vi "Reserve Coral.vi"(7 "Description":string="Reserve", 8 "Command Info":T1, 10 "Command Name":string) -> (0 "Command Info":T1)   [LabVIEW 2023]
uses:
  <vilib>/Rock Robotics/WPI/Framework/Command Status Info.ctl
  <vilib>/Rock Robotics/WPI/Framework/Completion Status.ctl
  <vilib>/Rock Robotics/WPI/Framework/Completion Notifier.ctl
  Implementation/Coral Setpoints.ctl
  Implementation/Coral Operations.ctl
  Support Code/Teleop Util/Coral States.ctl
  Support Code/Teleop Util/Scoring Levels.ctl
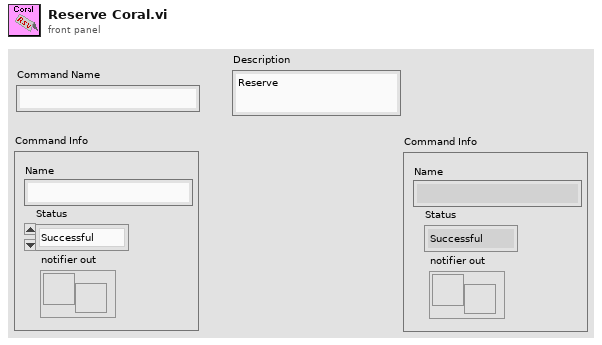
[diagram p1: front panel]
types:
  T1 = typedef "Command Status Info.ctl" = cluster{"Name":string, "Status":T2, "notifier out":T3}
  T2 = typedef "Completion Status.ctl" = enum16{"Successful", "Aborted", "Incomplete"}
  T3 = typedef "Completion Notifier.ctl" = refnum<notifier>
  T4 = typedef "Coral Setpoints.ctl" = cluster{"Operation":T5, "Coral States":T6, "Confirm or Negate":bool, "Positional Array":dbl[], "Setpoint State":T7}
  T5 = typedef "Coral Operations.ctl" = enum16{"Reserve", "Read Current", "Immediate", "Calibrate"}
  T6 = typedef "Coral States.ctl" = enum16{"Grounded", "Coral Intake", "Scoring Sequence", "Hold Position", "Score", "Manual Override", "Climb Safety Mode"}
  T7 = typedef "Scoring Levels.ctl" = enum16{"Trough", "L2", "L3", "L4", "Default"}
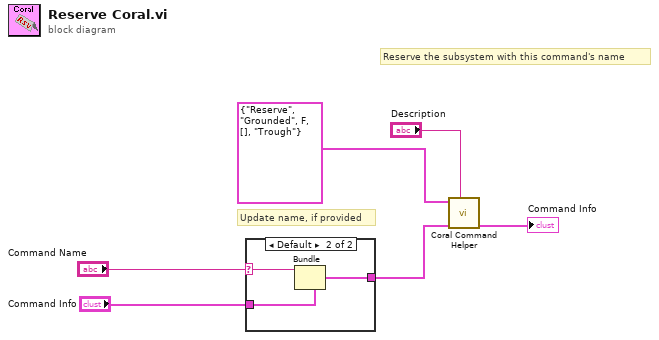
[diagram p0: block diagram]
diagram:
  # "Update name, if provided"
  # "Reserve the subsystem with this command's name"
  n1 = case shown="Default" "Command Name" {
    selector: "Command Name" -> [_ w8]
    tunnel: "Command Info" -> [w7 w10]
    tunnel: [w7 w9] -> w3
    frame "" {
    }
    frame Default {
      n2 = Bundle(cluster=w10, "Name"=w8) -> (w9:T1)  [unwired: 2 in]
    }
  }
  n3 = call "Coral Command Helper.vi"("Description"="Description", "Command Info In"=w3, "SubSystem Data"=T4 {"Operation"=enum."Reserve", "Coral States"=enum."Grounded", "Confirm or Negate"=FALSE, "Positional Array"=[], "Setpoint State"=enum."Trough"}) -> ("Command Info Out"=→"Command Info":T1)  [unwired: 6 in, 2 out]
